vi "ConfigureAcquisition.vi"(5 "Reference Level (dBm)":fxp<+/-,14,7>, 6 "Number of Samples":i32, 7 "Continuous":bool, 8 "error in (no error)":errorcluster, 9 "Center Frequency (Hz)":u32, 10 "Data Rate":T1 items=["320.000 kS/s (NI 9770)", "256.000 kS/s (NI 9770)", "128.000 kS/s (NI 9770)", "64.000 kS/s (NI 9770)", "32.000 kS/s (NI 9770)", "16.000 kS/s (NI 9770)", "8.000 kS/s (NI 9770)", "4.000 kS/s (NI 9770)"], 11 "9770 API in":refnum<class "9770 API.lvclass">) -> (0 "error out":errorcluster, 3 "9770 API out":refnum<class "9770 API.lvclass">)   [LabVIEW 2017, in "9770 API.lvclass"]
uses:
  <vilib>/addons/InsightCM/Devices/Shared/Emsa/Emsa9770API/9770 API.lvclass
  <vilib>/LabVIEW Targets/FPGA/cRIO/shared/nicrio_ModuleControls/nicrio_cRIO-9770_DataRatesRing.ctl
  <vilib>/addons/InsightCM/Devices/Shared/Emsa/Emsa9770API/9770 API.lvclass/9770 API.ctl
  <vilib>/Utility/error.llb/Error Cluster From Error Code.vi
  <vilib>/rvi/errors/niLvFpgaAdjustHostInterfaceError.vi
  <vilib>/rvi/interface/nirviReadWriteControl/nirviReadWriteControl.xnode
  <vilib>/addons/InsightCM/Devices/Shared/Emsa/Emsa9770API/controls/FPGATypeDef.ctl
  NiFpgaLv.dll
  <vilib>/rvi/interface/Simulation/niFpgaSimulationCallBeginRW.vi
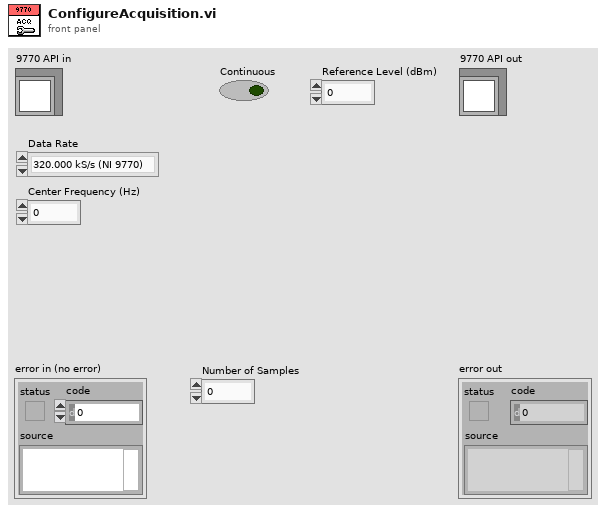
[diagram p1: front panel]
types:
  T1 = typedef "nicrio_cRIO-9770_DataRatesRing.ctl" = u8
  T2 = cluster{"Center Frequency (Hz)":u32, "Data Rate":u8, "Number of Samples":i32, "Continuous":bool, "Reference Level (dBm)":fxp<+/-,14,7>}
  T3 = typedef "9770 API.lvclass/FPGATypeDef.ctl" = refnum<k20>
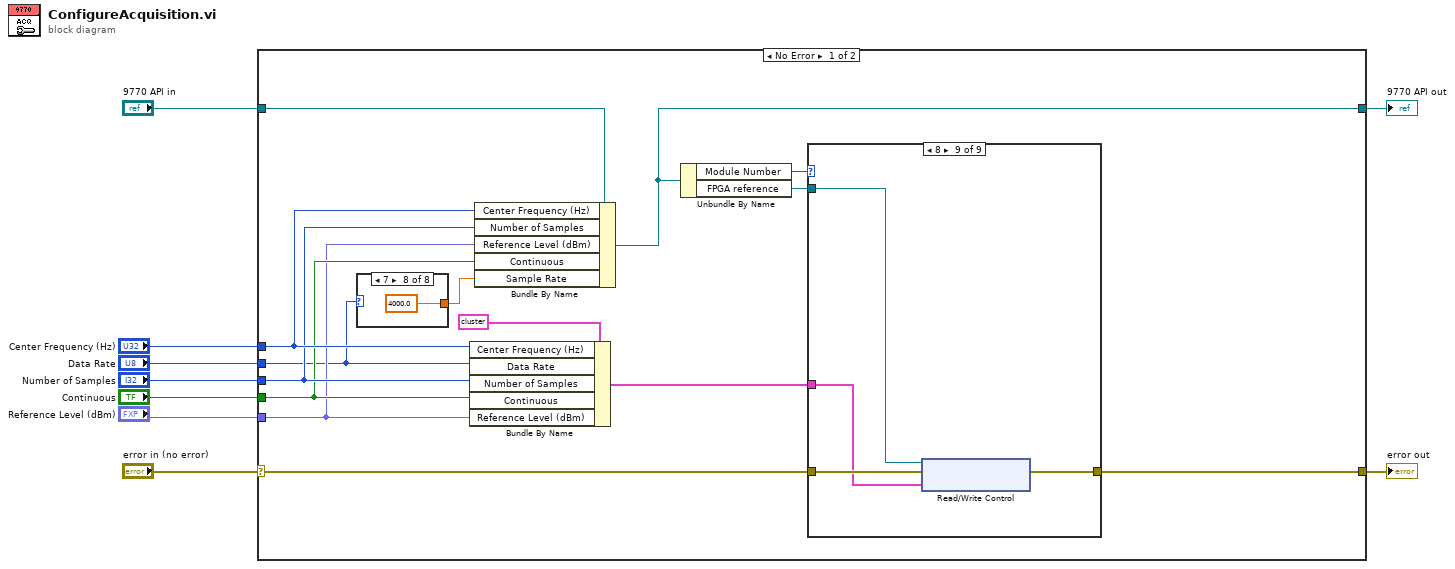
[diagram p0: block diagram]
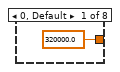
[diagram p2: hidden frame]
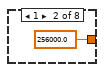
[diagram p3: hidden frame]
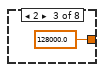
[diagram p4: hidden frame]
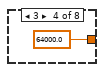
[diagram p5: hidden frame]
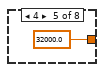
[diagram p6: hidden frame]
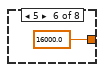
[diagram p7: hidden frame]
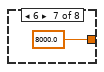
[diagram p8: hidden frame]
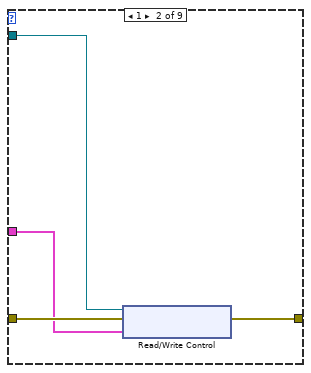
[diagram p10: hidden frame]
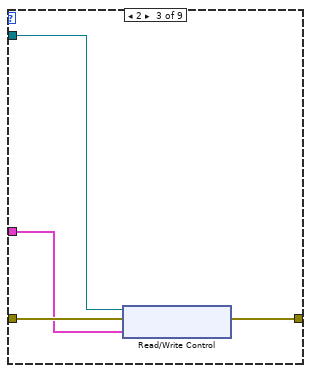
[diagram p11: hidden frame]
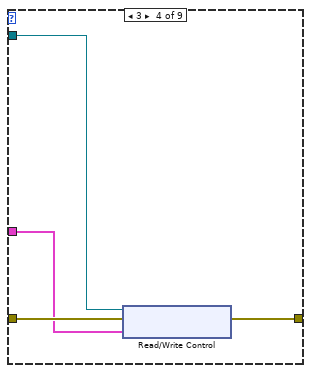
[diagram p12: hidden frame]
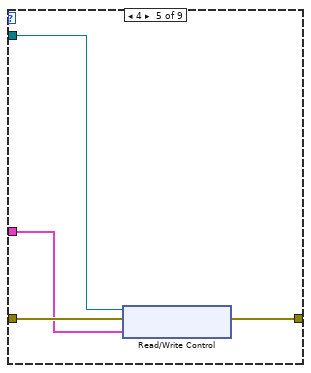
[diagram p13: hidden frame]
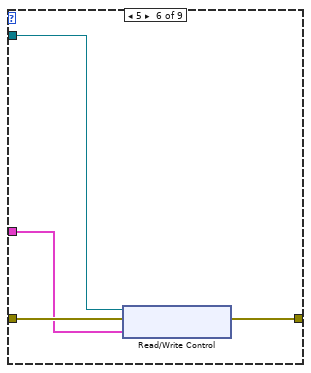
[diagram p14: hidden frame]
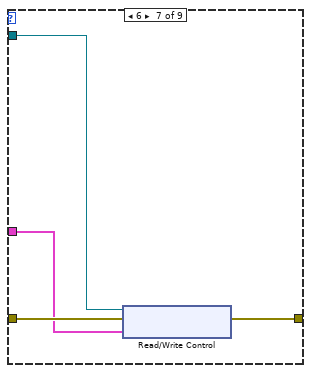
[diagram p15: hidden frame]
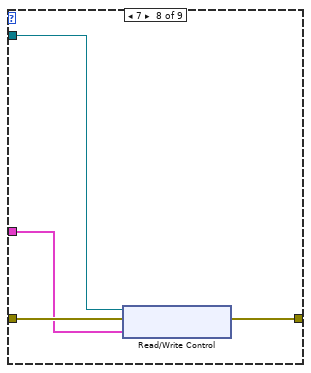
[diagram p16: hidden frame]
diagram:
  n1 = case shown="No Error" "error in (no error)" {
    selector: "error in (no error)" -> [w22 w66]
    tunnel: [w20 w66] -> w8
    tunnel: [w16 w65] -> w6
    tunnel: "9770 API in" -> [w17 w65]
    tunnel: "Center Frequency (Hz)" -> [w15 _]
    tunnel: "Data Rate" -> [w11 _]
    tunnel: "Number of Samples" -> [w14 _]
    tunnel: "Continuous" -> [w13 _]
    tunnel: "Reference Level (dBm)" -> [w12 _]
    frame No Error {
      n2 = case shown="7" w11 {
        tunnel: [320000.0 256000.0 128000.0 64000.0 32000.0 16000.0 8000.0 4000.0] -> w10
        frame 0, Default {
        }
        frame 1 {
        }
        frame 2 {
        }
        frame 3 {
        }
        frame 4 {
        }
        frame 5 {
        }
        frame 6 {
        }
        frame 7 {
        }
      }
      n3 = Bundle By Name(cluster=T2 {"Center Frequency (Hz)"=0, "Data Rate"=0, "Number of Samples"=0, "Continuous"=FALSE, "Reference Level (dBm)"=0.0} ("AcqSettings.Ch1"), "Center Frequency (Hz)"=w15, "Data Rate"=w11, "Number of Samples"=w14, "Continuous"=w13, "Reference Level (dBm)"=w12) -> (w18:T2)
      n4 = Bundle By Name(cluster=w17, "Center Frequency (Hz)"=w15, "Number of Samples"=w14, "Reference Level (dBm)"=w12, "Continuous"=w13, "Sample Rate"=w10) -> (w16:refnum<class "9770 API.lvclass">)
      n5 = Unbundle By Name(w16) -> ("Module Number"=w23:u32, "FPGA reference"=w21:T3)
      n6 = case shown="8" w23 {
        tunnel: w22 -> [w32 w36 w40 w44 w48 w52 w56 w60 w64]
        tunnel: w21 -> [_ w35 w39 w43 w47 w51 w55 w59 w63]
        tunnel: [w32 w34 w38 w42 w46 w50 w54 w58 w62] -> w20
        tunnel: w18 -> [_ w33 w37 w41 w45 w49 w53 w57 w61]
        frame 0, Default {
        }
        frame 1 {
          n7 = xnode "Read/Write Control"("FPGA VI Reference In"=w35, "error in"=w36, "AcqSettings.Ch 1"=w33) -> ("error out"=w34:errorcluster)  [unwired: 1 out]
        }
        frame 2 {
          n8 = xnode "Read/Write Control"("FPGA VI Reference In"=w39, "error in"=w40, "AcqSettings.Ch 2"=w37) -> ("error out"=w38:errorcluster)  [unwired: 1 out]
        }
        frame 3 {
          n9 = xnode "Read/Write Control"("FPGA VI Reference In"=w43, "error in"=w44, "AcqSettings.Ch 3"=w41) -> ("error out"=w42:errorcluster)  [unwired: 1 out]
        }
        frame 4 {
          n10 = xnode "Read/Write Control"("FPGA VI Reference In"=w47, "error in"=w48, "AcqSettings.Ch 4"=w45) -> ("error out"=w46:errorcluster)  [unwired: 1 out]
        }
        frame 5 {
          n11 = xnode "Read/Write Control"("FPGA VI Reference In"=w51, "error in"=w52, "AcqSettings.Ch 5"=w49) -> ("error out"=w50:errorcluster)  [unwired: 1 out]
        }
        frame 6 {
          n12 = xnode "Read/Write Control"("FPGA VI Reference In"=w55, "error in"=w56, "AcqSettings.Ch 6"=w53) -> ("error out"=w54:errorcluster)  [unwired: 1 out]
        }
        frame 7 {
          n13 = xnode "Read/Write Control"("FPGA VI Reference In"=w59, "error in"=w60, "AcqSettings.Ch 7"=w57) -> ("error out"=w58:errorcluster)  [unwired: 1 out]
        }
        frame 8 {
          n14 = xnode "Read/Write Control"("FPGA VI Reference In"=w63, "error in"=w64, "AcqSettings.Ch 8"=w61) -> ("error out"=w62:errorcluster)  [unwired: 1 out]
        }
      }
    }
    frame Error {
    }
  }
  "error out" <- w8
  "9770 API out" <- w6
